vi "Wheel Speed Filter.vi"(1 "Smoothing Factor (0-1)":dbl=0.02, 2 "Previous Wheel Speed":i16, 3 "Wheel Speed":i16) -> (0 "Smoothed Wheel Speed":i16)   [LabVIEW 2013]
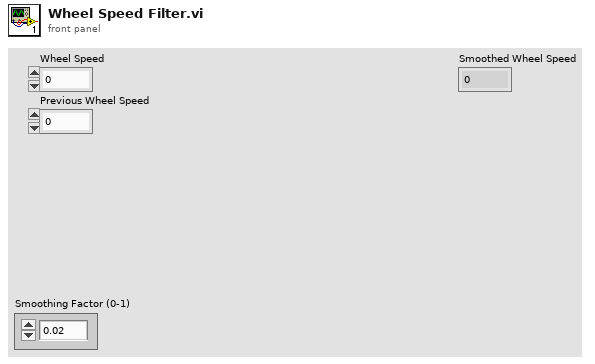
[diagram p1: front panel]
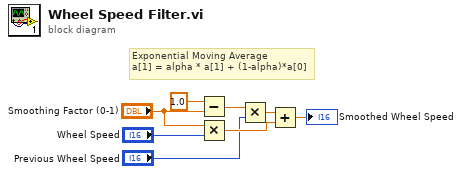
[diagram p0: block diagram]
diagram:
  # "Exponential Moving Average\na[1] = alpha * a[1] + (1-alpha)*a[0]"
  n1 = Subtract(x=1.0, y="Smoothing Factor (0-1)") -> (x-y=w4:dbl)
  n2 = Multiply(x="Smoothing Factor (0-1)", y="Wheel Speed") -> (x*y=w6:dbl)
  n3 = Multiply(x=w4, y="Previous Wheel Speed") -> (x*y=w5:dbl)
  n4 = Add(x=w5, y=w6) -> (x+y=→"Smoothed Wheel Speed":dbl)
